vi "LibXML_SetContent.vi"(8 "error in (no error)":errorcluster, 10 "content":string, 11 "node":u32) -> (0 "error out":errorcluster, 3 "node copy":u32)   [LabVIEW 2019, in "Tools.lvlib" / "LibXML.lvlib"]
doc: "Function: xmlNodeSetContent\n\nvoid xmlNodeSetContent (xmlNodePtr cur, \n const xmlChar * content)\n\nReplace the content of a node.\ncur: the node being modified\ncontent: the new value of the content"
uses:
  LibXML.lvlib
  dll/libxml2.dll
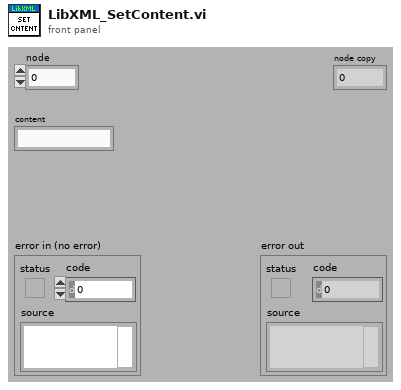
[diagram p1: front panel]
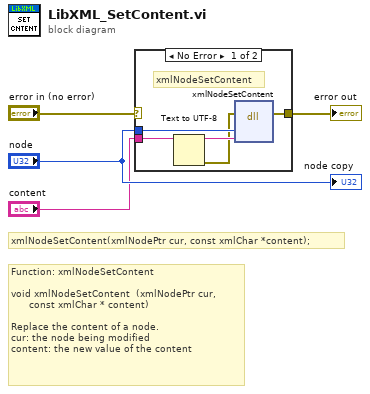
[diagram p0: block diagram]
diagram:
  # "Function: xmlNodeSetContent\n\nvoid\txmlNodeSetContent\t\t(xmlNodePtr cur, \n\t\t\t\t\t const xmlChar * content)\n\nReplace the content of a node.\ncur:\tthe node being modified\ncontent:\tthe new value of the content"
  # "xmlNodeSetContent(xmlNodePtr cur, const xmlChar *content);"
  n1 = case shown="No Error" "error in (no error)" {
    selector: "error in (no error)" -> [_ w10]
    tunnel: [w8 w10] -> w3
    tunnel: "node" -> [w9 _]
    tunnel: "content" -> [w7 _]
    frame No Error {
      # "xmlNodeSetContent"
      n2 = Text to UTF-8(11:w7) -> (0:w5:errorcluster, 3:w6:string)  [unwired: 2 in]
      n3 = dll-call lib="C:/Projects/_Prywatne/MyCIT/Framework/Tools/XML/LibXML/dll/libxml2.dll" fn="xmlNodeSetContent"(error in=w5, "node"=w9, "content"=w6) -> (error out=w8:errorcluster)  [unwired: 5 in, 1 out]
    }
    frame Error {
    }
  }
  "error out" <- w3
  "node copy" <- "node"
